vi "Day1_integer.vi"() -> ()   [LabVIEW 2014]
panel:
  out "x-y*floor(x/y)":u32
  out "floor(x/y)":u32
  in  "숫자형 4":u32
  out "y":dbl
  in  "숫자형 3":dbl
  out "숫자형 2":u32
  in  "링":u32(ring) items=["Second"=1, "No of seconds in minute"=60, "No of seconds in hour"=3600, "Seconds in a Day"=864000]
  out "색 상자":u32(colorbox)
  in  "숫자형":T1 format="%.0x"
  out "x+y":i8
  in  "i8 2":i8
  in  "i8":i8
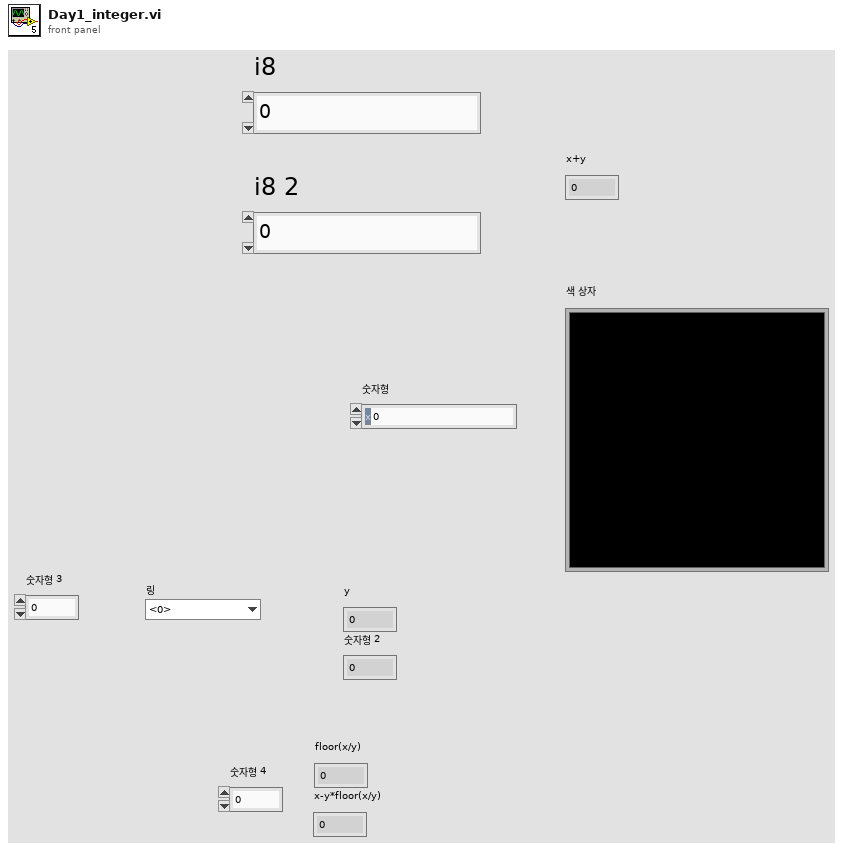
[diagram p1: front panel]
types:
  T1 = typedef "컨트롤 2.ctl" = i32
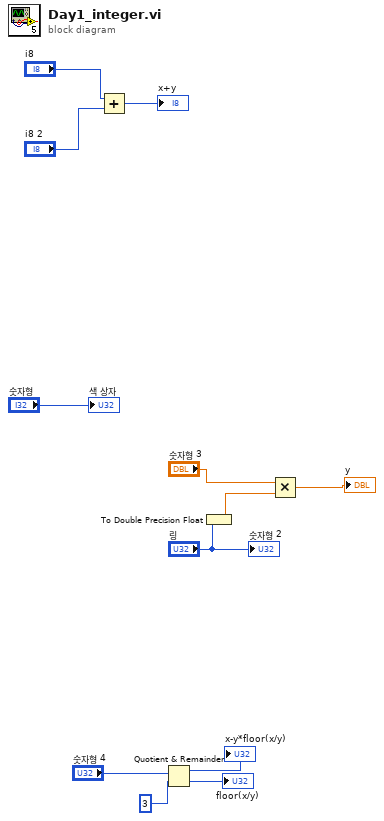
[diagram p0: block diagram]
diagram:
  n1 = Add(x="i8", y="i8 2") -> (x+y=→"x+y":i8)
  n2 = Quotient & Remainder(x="숫자형 4", y=u32 3 ("floor(x/y)")) -> (x-y*floor(x/y)=→"x-y*floor(x/y)":u32, floor(x/y)=→"floor(x/y)":u32)
  n3 = To Double Precision Float(number="링") -> (double precision float=w6:dbl)
  n4 = Multiply(x="숫자형 3", y=w6) -> (x*y=→"y":dbl)
  "색 상자" <- "숫자형"
  "숫자형 2" <- "링"
